vi "Begin.vi"(8 "error in":errorcluster) -> (0 "error out":errorcluster)   [LabVIEW 2014]
doc: "Called before other user functions, this VI is expected to open initial I/O refnums, load in file data, and do all program initialization. Notice that the <B>error out</B> terminal is simply used for data flow. Wiring it to other structures or subVIs ensures that this VI runs first."
uses:
  <vilib>/Rock Robotics/WPI/DriverStation/WPI_DriverStationRobotMode2.ctl
  Robot Global Data.vi
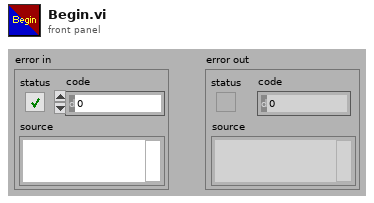
[diagram p1: front panel]
types:
  T1 = typedef "WPI_DriverStationRobotMode2.ctl" = enum16{"Autonomous Disabled", "Autonomous Enabled", "Teleop Disabled", "Teleop Enabled", "Disconnected", "Finish", "Test Disabled", "Test Enabled", "Emergency Stopped"}
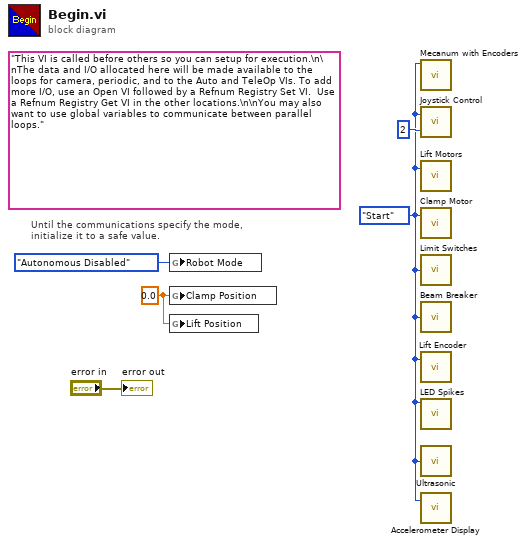
[diagram p0: block diagram]
diagram:
  w2 = 0.0 ("Clamp Position")
  w1 = enum8{"Start", "Run", "Finish"}."Start" ("Mode")
  (unwired) "This VI is called before others so you can setup for execution.\n\nThe data and I/O allocated here will be made available to the loops for camera, periodic, and to the Auto and TeleOp VIs. To add more I/O, use an Open VI followed by a Refnum Registry Set VI.  Use a Refnum Registry Get VI in the other locations.\n\nYou may also want to use global variables to communicate between parallel loops."
  # "Until the communications specify the mode,\ninitialize it to a safe value."
  n1 = global write "Robot Global Data.vi" "Robot Mode"(WPI_DriverStationRobotMode2."Autonomous Disabled" ("Robot Mode")) -> ()
  n2 = global write "Robot Global Data.vi" "Clamp Position"(w2) -> ()
  n3 = global write "Robot Global Data.vi" "Lift Position"(w2) -> ()
  n4 = call "Mecanum with Encoders.vi"("Mode"=w1) -> ()  [unwired: 9 in, 1 out]
  n5 = call "Joystick Control.vi"("Number of Joysticks"=2, "Mode"=w1) -> ()  [unwired: 1 out]
  n6 = call "Lift Motors.vi"("Mode"=w1) -> ()  [unwired: 2 in]
  n7 = call "Clamp Motor.vi"("Mode"=w1) -> ()  [unwired: 2 in]
  n8 = call "Limit Switches.vi"("Mode"=w1) -> ()  [unwired: 1 out]
  n9 = call "Beam Breaker.vi"("Mode"=w1) -> ()  [unwired: 1 in, 1 out]
  n10 = call "Lift Encoder.vi"("Mode"=w1) -> ()  [unwired: 1 in, 1 out]
  n11 = call "LED Spikes.vi"("Mode"=w1) -> ()  [unwired: 3 in]
  n12 = call "Ultrasonic.vi"("Mode"=w1) -> ()  [unwired: 1 out]
  n13 = call "Accelerometer Display.vi"("Mode"=w1) -> ()  [unwired: 1 in, 1 out]
  "error out" <- "error in"
